vi "FG Battery Voltage.vi"(1 "FG Action":T1, 2 "Battery Voltage in":dbl) -> (0 "Battery Voltage out":dbl)   [LabVIEW 2009]
uses:
  Actions for FG's.ctl
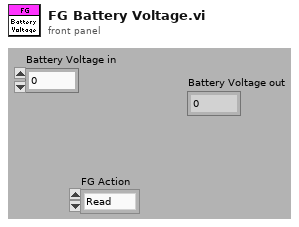
[diagram p1: front panel]
types:
  T1 = typedef "Actions for FG's.ctl" = enum16{"Read", "Write"}
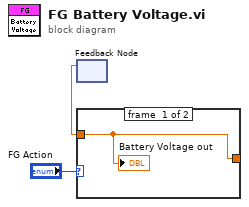
[diagram p0: block diagram]
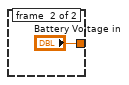
[diagram p2: hidden frame]
diagram:
  n1 = feedback #1() -> (w1:dbl)  [unwired: 1 in]
  n2 = case shown="\"Read\", Default" "FG Action" {
    tunnel: w1 -> [w4 _]
    tunnel: [w4 "Battery Voltage in"] -> w2
    frame #0 {
      "Battery Voltage out" <- w4
    }
    frame #1 {
    }
  }
